vi "Get Data - 複製.vi"() -> (0 "String":string, 1 "X10~X17":bool[](array[boolean]), 2 "X0~X7":bool[](array[boolean]), 3 "VISA Output":refnum<visa-resource-name>)   [LabVIEW 2009]
uses:
  <vilib>/Instr/_visa.llb/VISA Configure Serial Port (Instr).vi
panel:
  in  "COM Port":refnum<visa-resource-name>="COM3"
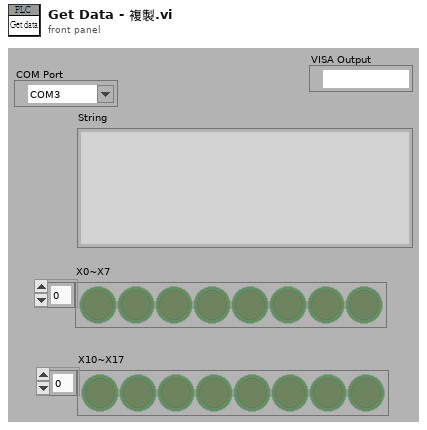
[diagram p1: front panel]
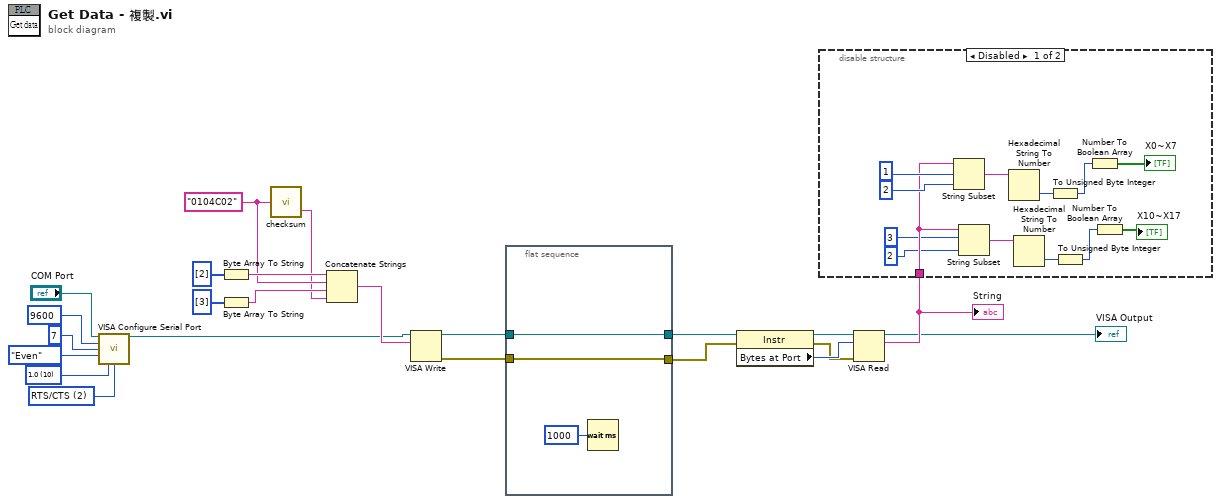
[diagram p0: block diagram]
diagram:
  w3 = u16 2 items=["None", "XON/XOFF", "RTS/CTS", "XON/XOFF & RTS/CTS", "DTR/DSR", "XON/XOFF & DTR/DSR"] ("flow control (0:none)")
  w4 = u16 10 items=["1.0"=10, "1.5"=15, "2.0"=20] ("stop bits (10: 1 bit)")
  w12 = "0104C02"
  n1 = call-poly "VISA Configure Serial Port"("VISA resource name"="COM Port", "baud rate (9600)"=u32 9600, "data bits (8)"=u16 7, "parity (0:none)"=enum16{"None", "Odd", "Even", "Mark", "Space"}."Even", "stop bits (10: 1 bit)"=w4, "flow control (0:none)"=w3) -> ("VISA resource name out"=w1:refnum<visa-resource-name>)  [unwired: 8 in, 1 out]
  n2 = Byte Array To String(unsigned byte array=u8[] [2]) -> (string=w21:string)
  n3 = Byte Array To String(unsigned byte array=u8[] [3]) -> (string=w13:string)
  n4 = call "checksum.vi"("Data"=w12) -> ("Check Sum"=w11:string)  [unwired: 2 in, 1 out]
  n5 = Concatenate Strings(w21, w12, w13, w11) -> (w10:string)
  n6 = VISA Write(VISA resource name=w1, write buffer=w10) -> (VISA resource name out=w20:refnum<visa-resource-name>, error out=w19:errorcluster)  [unwired: 1 in, 1 out]
  n7 = flat-sequence {
    tunnel: [w25] -> w18
    tunnel: w20 -> [w25]
    tunnel: [w24] -> w17
    tunnel: w19 -> [w24]
    frame #0 {
      n8 = Wait (ms)(milliseconds to wait=u32 1000) -> ()  [unwired: 1 out]
    }
  }
  n9 = property class="Instr"(reference=w18, error in=w17) -> (reference out=w16:refnum<visa-resource-name>, error out=w14:errorcluster, "Bytes at Port"=w15:u32)
  n10 = VISA Read(VISA resource name=w16, byte count=w15, error in (no error)=w14) -> (VISA resource name out=→"VISA Output":refnum<visa-resource-name>, read buffer=w9:string)  [unwired: 2 out]
  "String" <- w9
  n11 = disable-structure shown="Disabled" {
    disable-tunnel: w9 -> [w30 _]
    frame #0 {
      n12 = String Subset(string=w30, offset (0)=1, length (rest)=2 ("length (rest)")) -> (substring=w36:string)
      n13 = String Subset(string=w30, offset (0)=3, length (rest)=2 ("length (rest)")) -> (substring=w31:string)
      n14 = Hexadecimal String To Number(string=w36) -> (number=w35:u32)  [unwired: 2 in, 1 out]
      n15 = Hexadecimal String To Number(string=w31) -> (number=w32:u32)  [unwired: 2 in, 1 out]
      n16 = To Unsigned Byte Integer(number=w35) -> (unsigned 8bit integer=w34:u8)
      n17 = To Unsigned Byte Integer(number=w32) -> (unsigned 8bit integer=w33:u8)
      n18 = Number To Boolean Array(number=w34) -> (Boolean array=→"X0~X7":bool[])
      n19 = Number To Boolean Array(number=w33) -> (Boolean array=→"X10~X17":bool[])
    }
    frame #1 {
    }
  }
